vi "纳清DO电极校准.vi"() -> ()   [LabVIEW 2016, in "斯坦道多参数.lvlib"]
uses:
  <vilib>/Utility/miscctls.llb/LVPointTypeDef.ctl
  <vilib>/Analysis/NI_AALBase.lvlib
  <vilib>/ptbypt/NI_PtbyPt.lvlib
panel:
  out "标液2":string="饱和标准液"
  out "标液1":string="零点标准液"
  out "第二点信号值":dbl
  out "第一点信号值":dbl
  out "盐度":sgl format="%#.2f"
  out "大气压力":sgl format="%#.2f"
  out "饱和值":sgl format="%#.2f"
  out "报警信息":string
  out "通讯状态":string
  out "第二点校准值":dbl
  out "第一点校准值":dbl
  in  "校准停止":bool
  in  "校准启动":bool
  in  "校准模式":enum16{"两点校准", "单点校准"}(ring)=enum."单点校准"
  out "最小值":sgl format="%#.2f"
  out "最大值":sgl format="%#.2f"
  out "波形图表":dbl(graph) caption="历史曲线"
  out "mean":dbl caption="均值" format="%#.2f"
  out "standard deviation":dbl caption="标准差" format="%#.2f"
  out "变异系数":dbl format="%#.6f"
  out "测量值":sgl format="%#.2f"
  out "提示":string
  out "原始光强数值":sgl caption="信号值" format="%#.6f"
  out "温度":dbl format="%#.2f"
  # "DO电极设定"
  # "℃"
  # "mg/L"
  # "%"
  # "nA"
  # "kPa"
  # "ppt"
  # "请选择校准模式:"
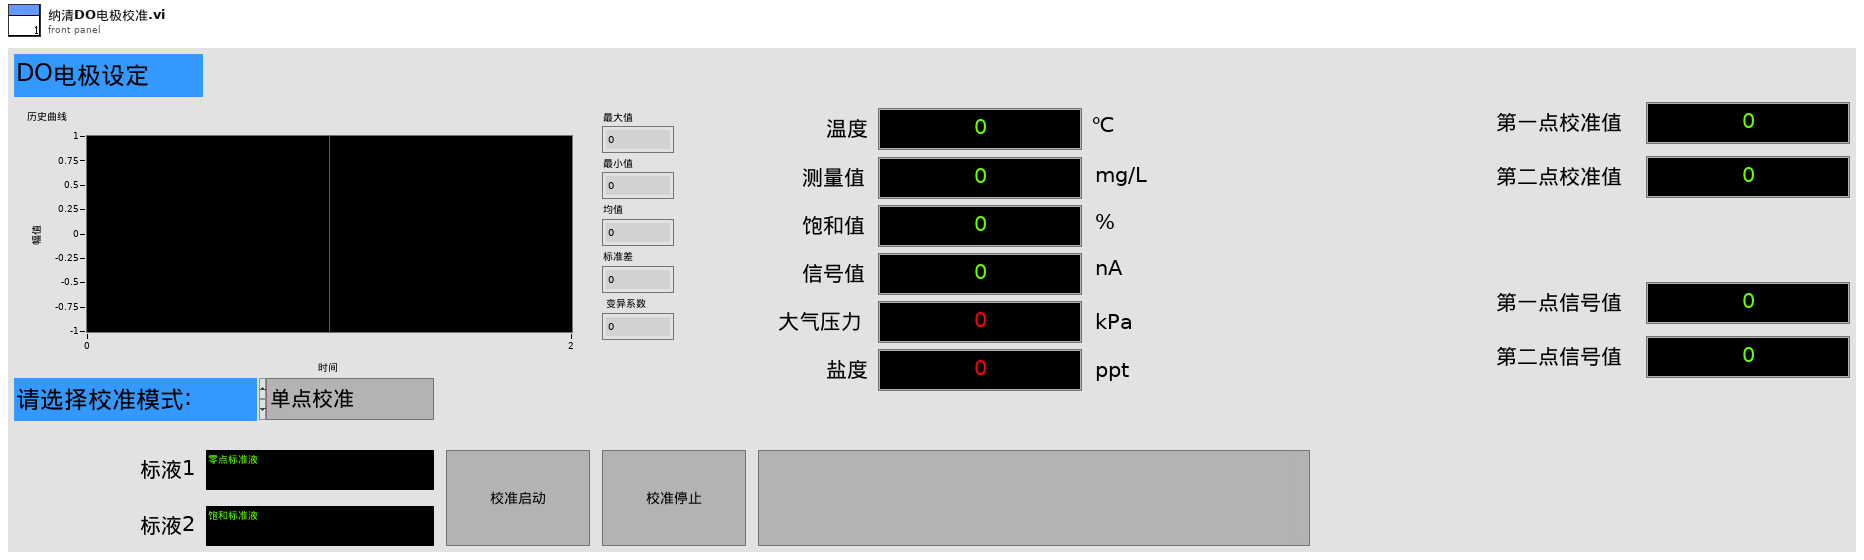
[diagram p1: front panel]
types:
  T1 = typedef "LVPointTypeDef.ctl" = cluster{"Horizontal":i16, "Vertical":i16}
  T2 = cluster{"报警码":u16, "溶解氧数值（mg/L）":sgl, "溶解氧数据（%）":sgl, "温度数据":sgl, "溶解氧原始信号 nA":sgl, "大气压力":sgl, "盐度":sgl, "0X0009_NC":string, "产品名称":string, "序列号":string, "硬件版本":string, "软件版本":string, "通讯地址":u16, "波特率":u16, "设备类型":u16, "0X0026_NC":string, "第一点原始数据":sgl, "第一点校准数据":sgl, "第二点原始数据":sgl, "第二点校准数据":sgl, "探头校准命令":u16, "温度校准参数":sgl, "温度校准命令":u16}
  T3 = enum8{"Enabled", "Disabled", "Disabled and Grayed Out"}
  T4 = cluster{"报警码":u16, "溶解氧数值（mg/L）":sgl, "溶解氧数据（%）":sgl, "温度数据":sgl, "溶解氧原始信号 nA":sgl, "大气压力":sgl, "盐度":sgl, "0X0009_NC":string, "产品名称":string, "序列号":string, "硬件版本":string, "软件版本":string, "通讯地址":u16, "波特率":u16, "设备类型":u16, "0X0026_NC":string, "第一点原始数据":sgl, "0X0033 NC":sgl, "第二点原始数据":sgl, "0X0037 NC":sgl, "探头校准命令":u16, "温度校准参数":sgl, "温度校准命令":u16}
  T5 = cluster{"ph":bool, "DO":bool, "Cond":bool, "Turb":bool, "叶绿素a":bool, "藻密度":bool, "ORP":bool}
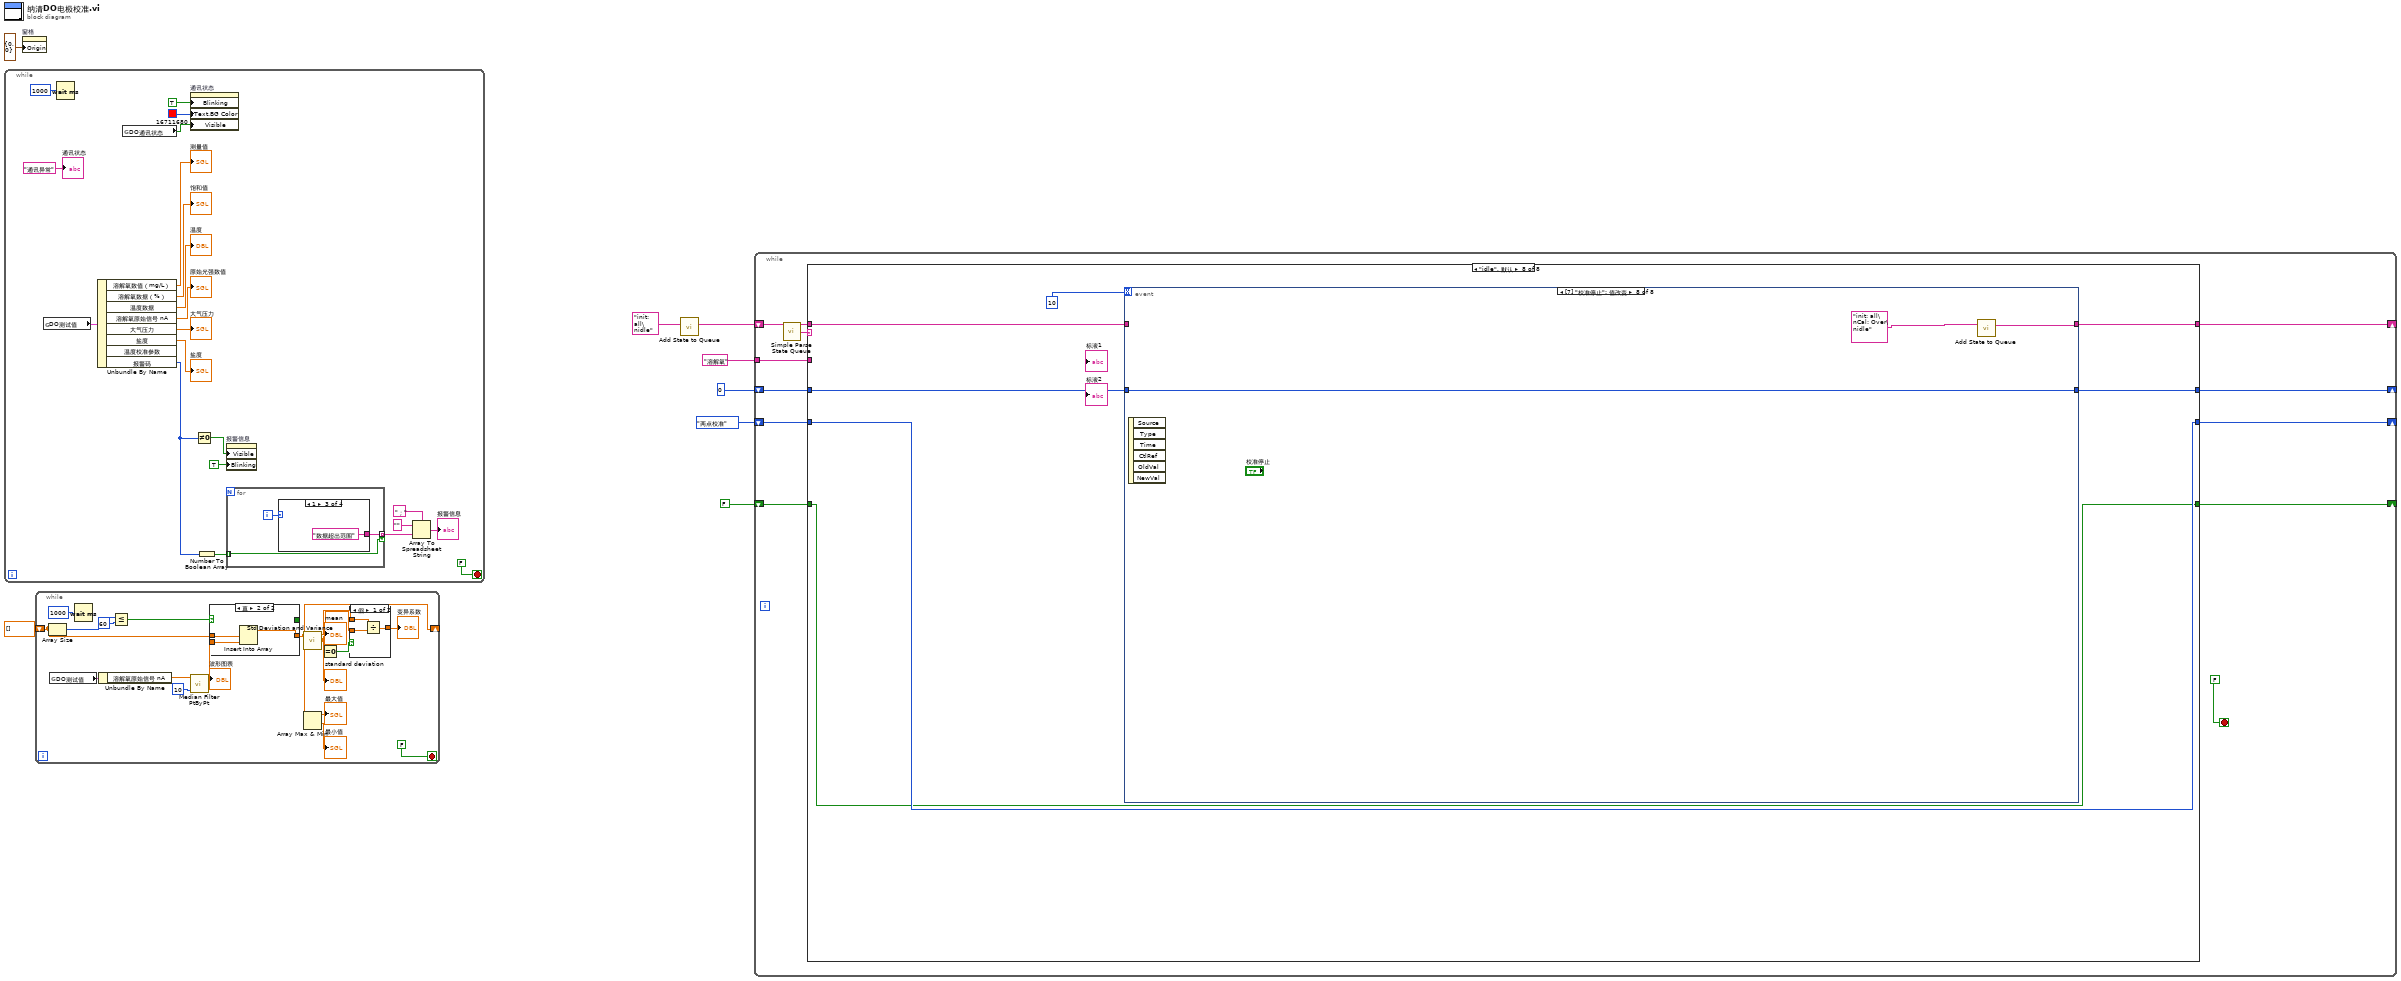
[diagram p0: block diagram]
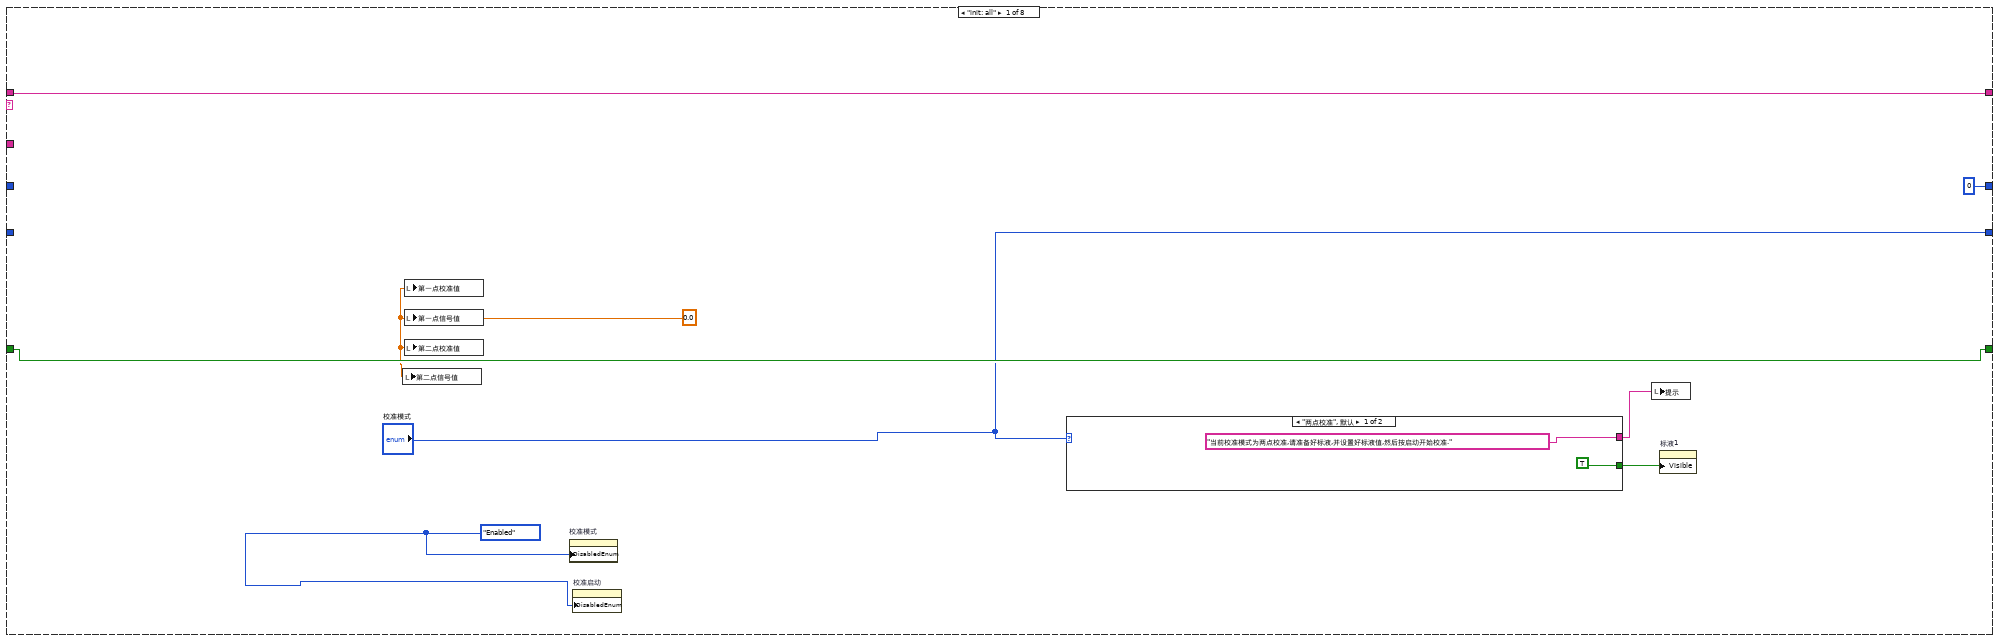
[diagram p2: hidden frame]
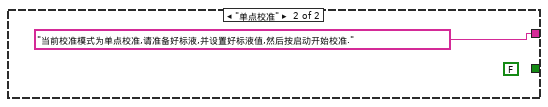
[diagram p3: hidden frame]
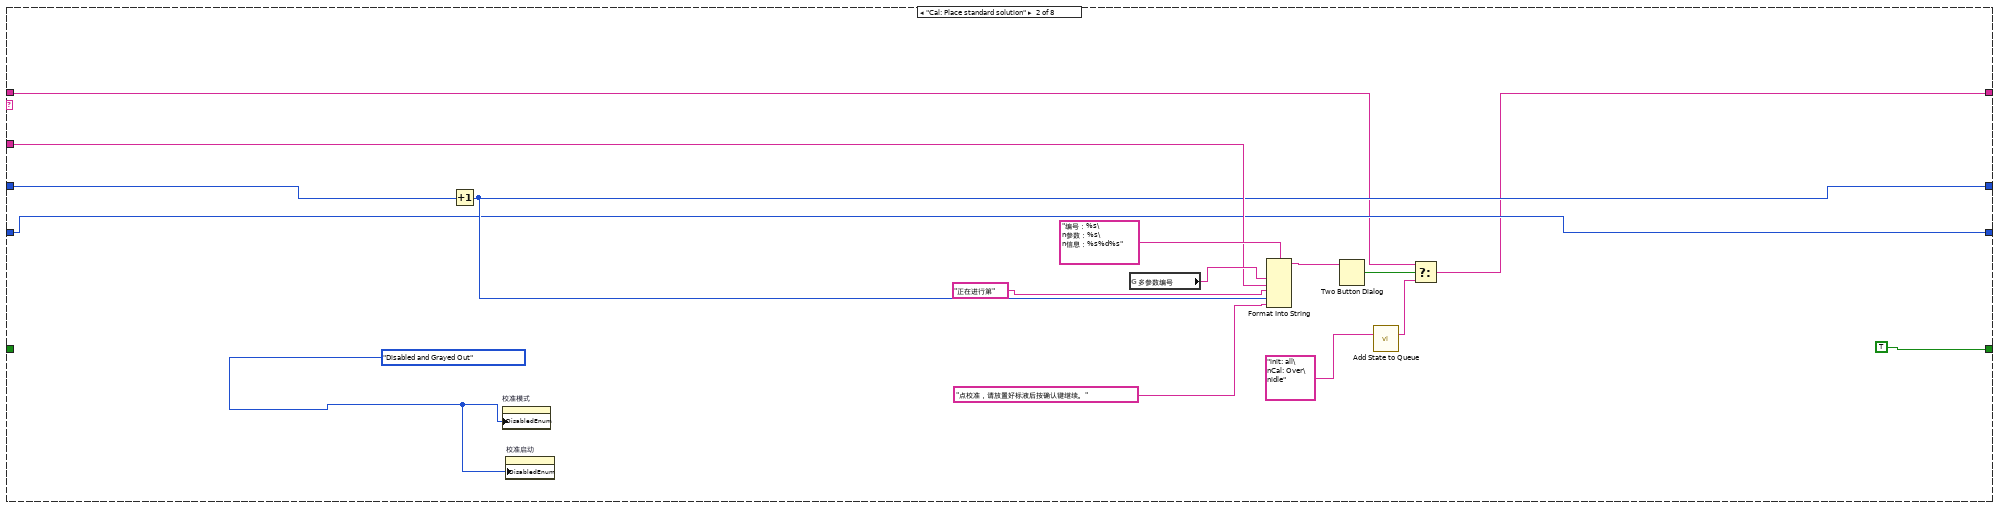
[diagram p4: hidden frame]
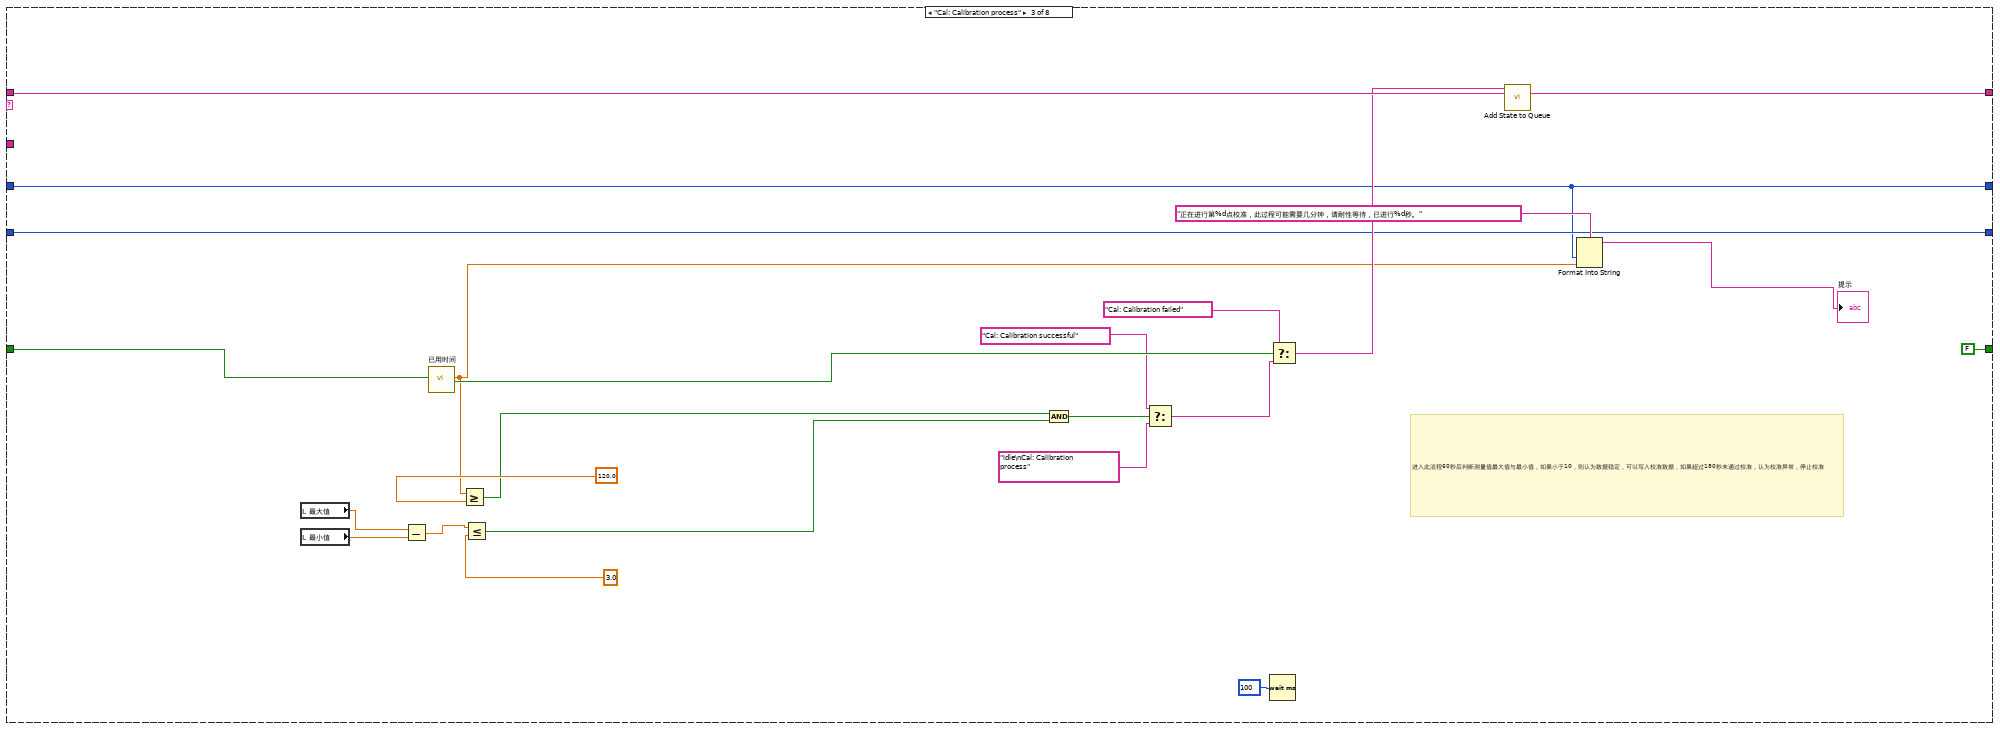
[diagram p5: hidden frame]
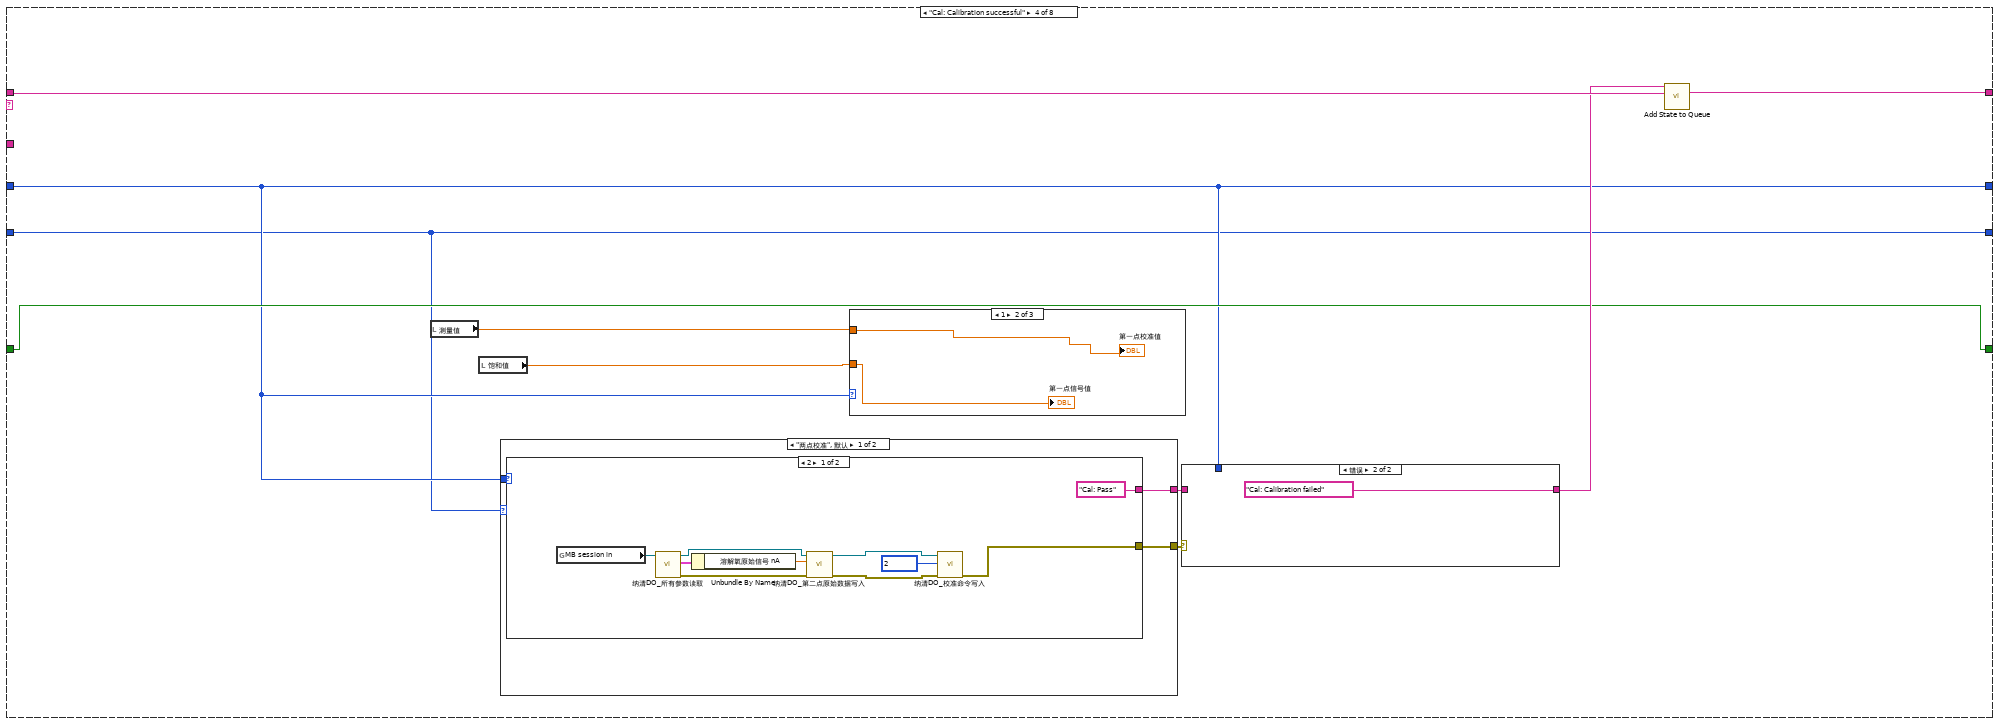
[diagram p6: hidden frame]
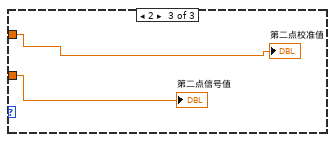
[diagram p8: hidden frame]
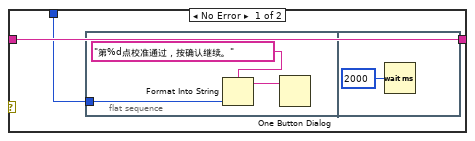
[diagram p9: hidden frame]
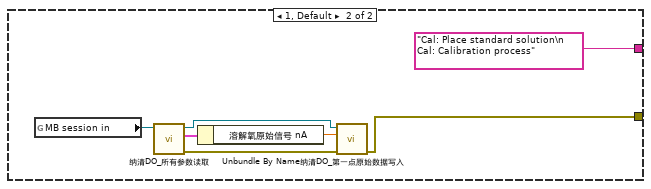
[diagram p10: hidden frame]
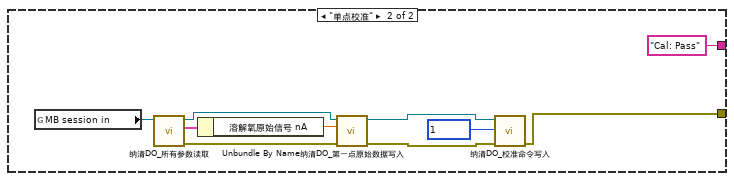
[diagram p11: hidden frame]
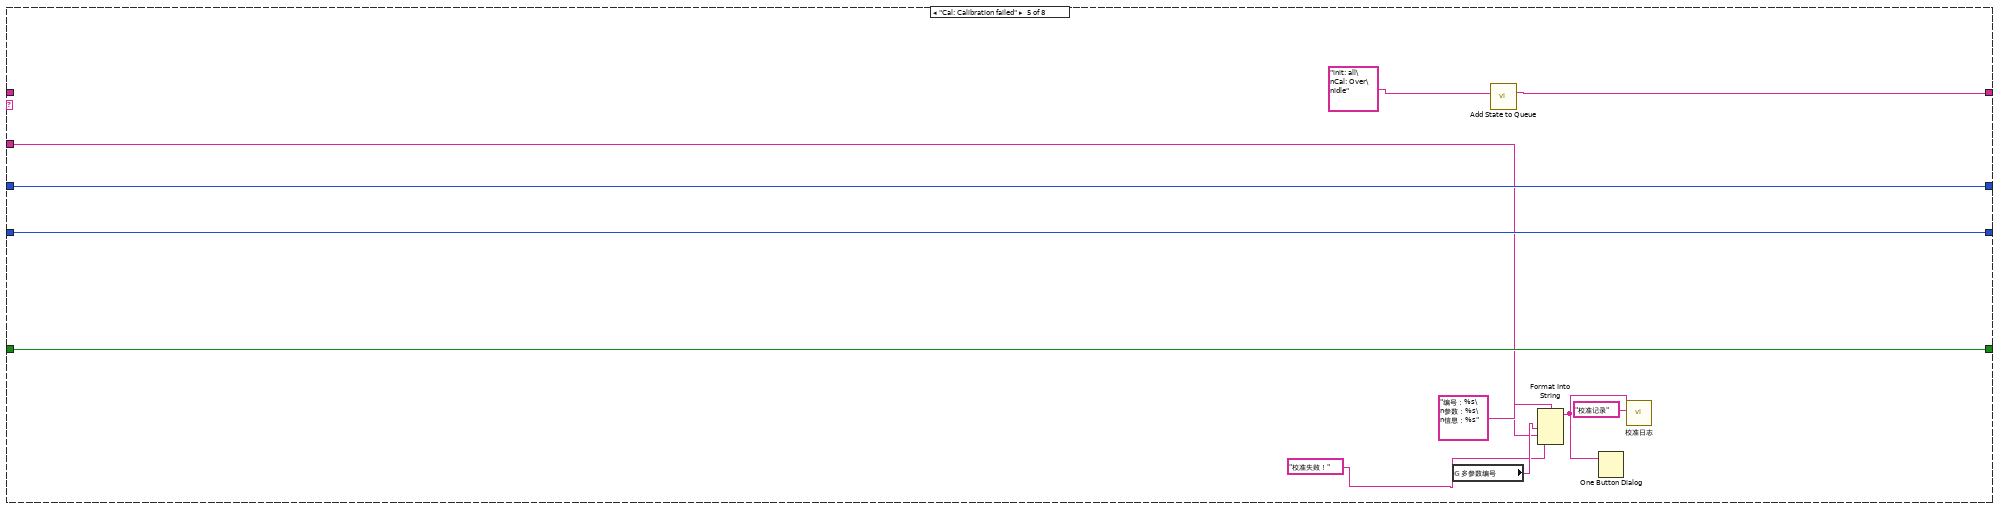
[diagram p12: hidden frame]
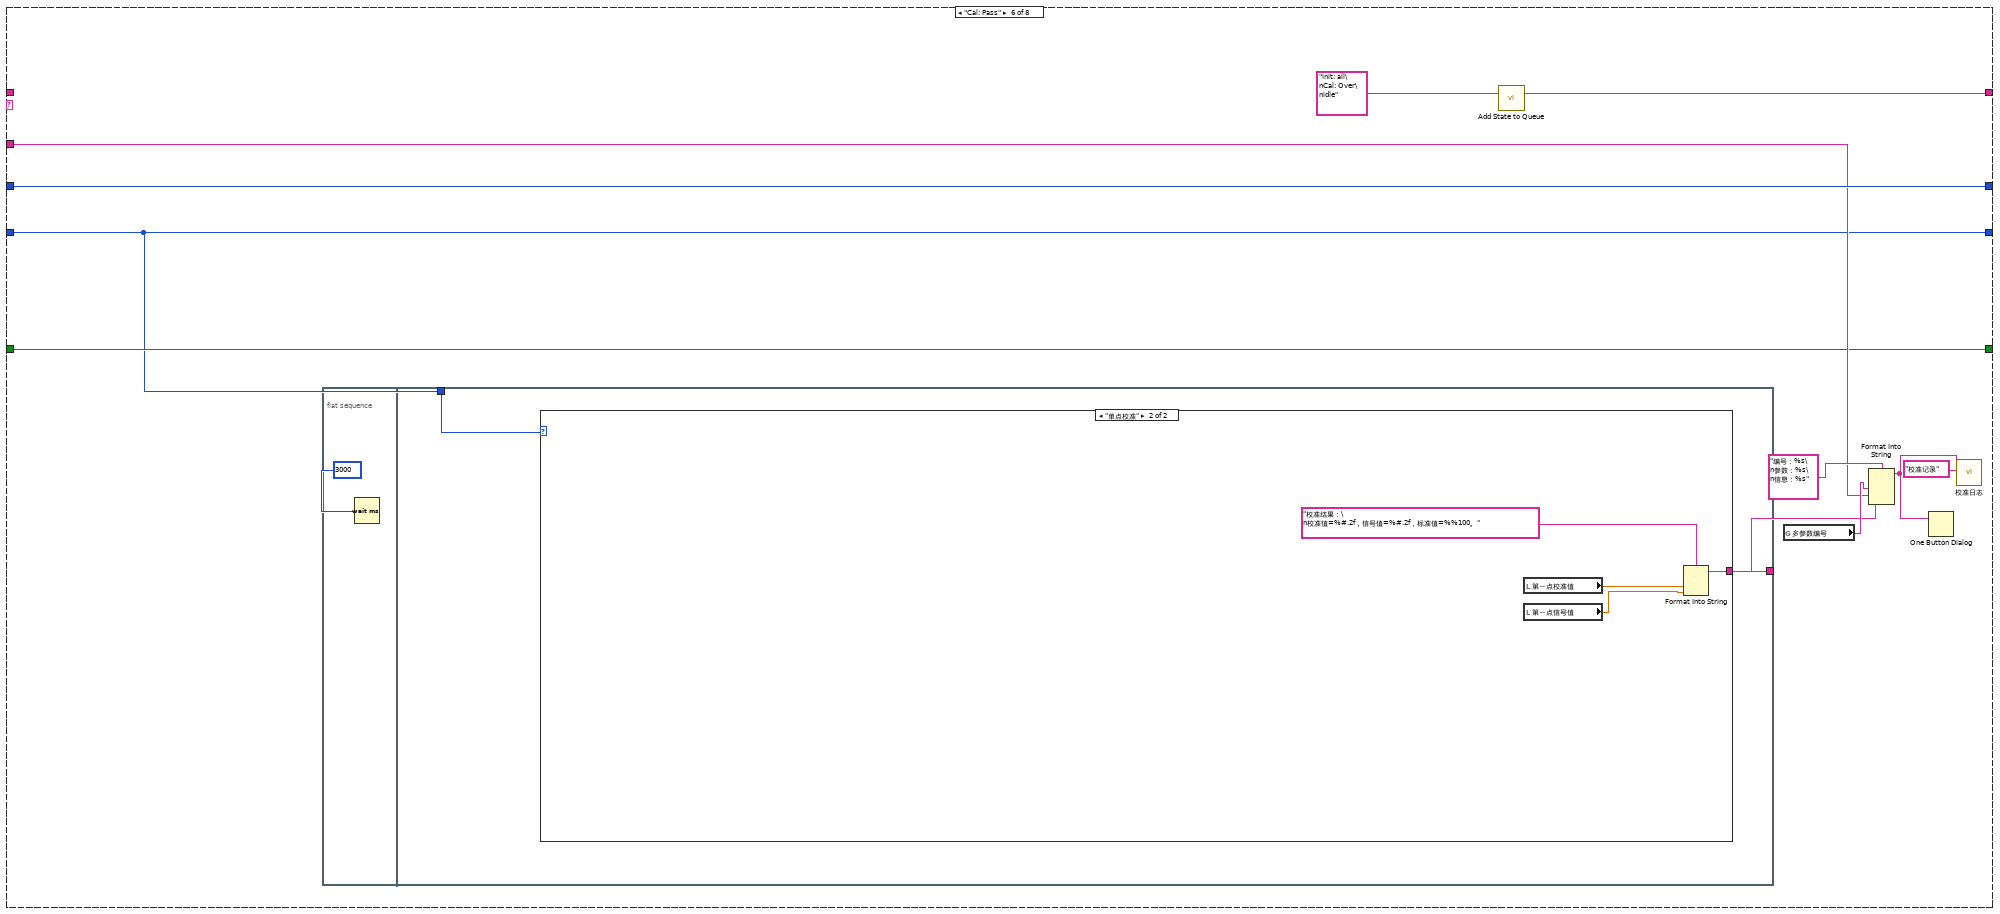
[diagram p13: hidden frame]
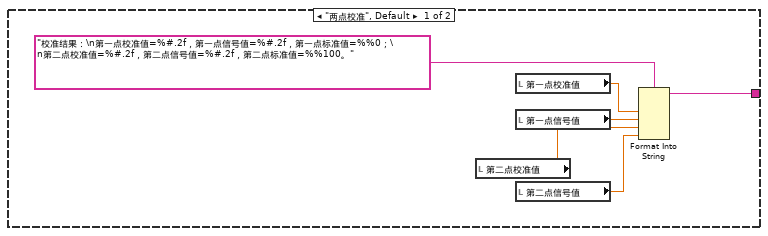
[diagram p14: hidden frame]
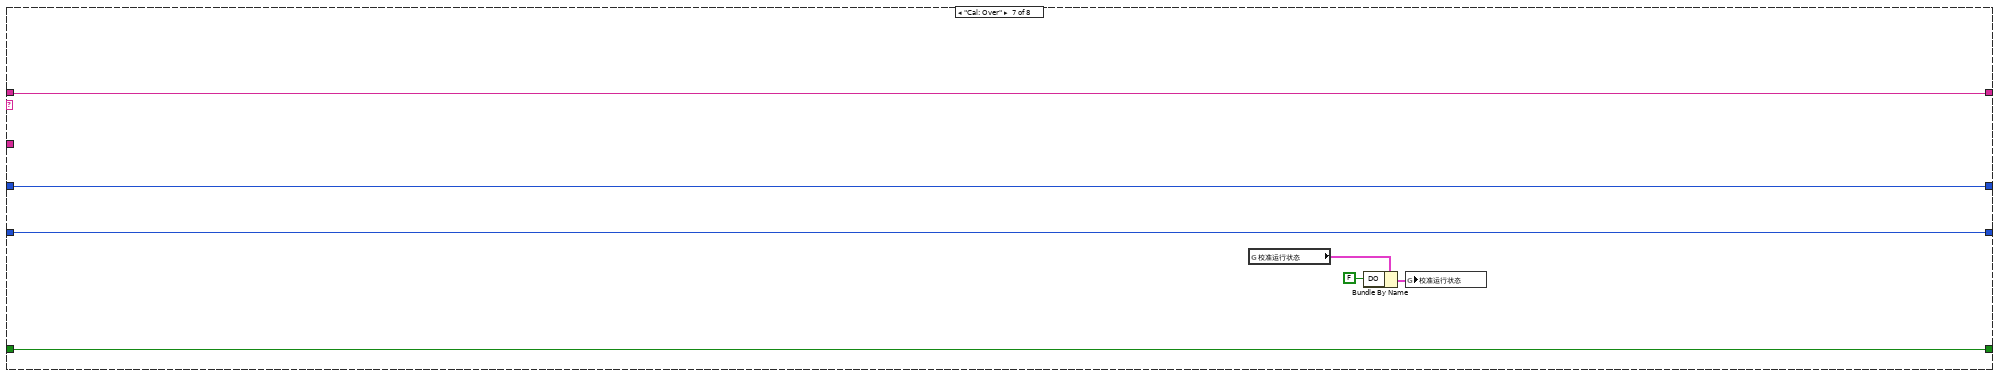
[diagram p15: hidden frame]
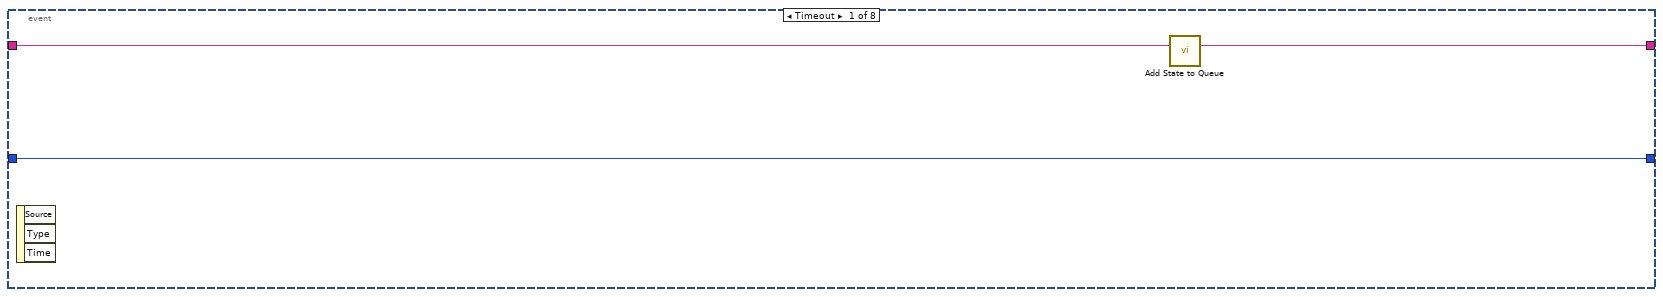
[diagram p16: hidden frame]
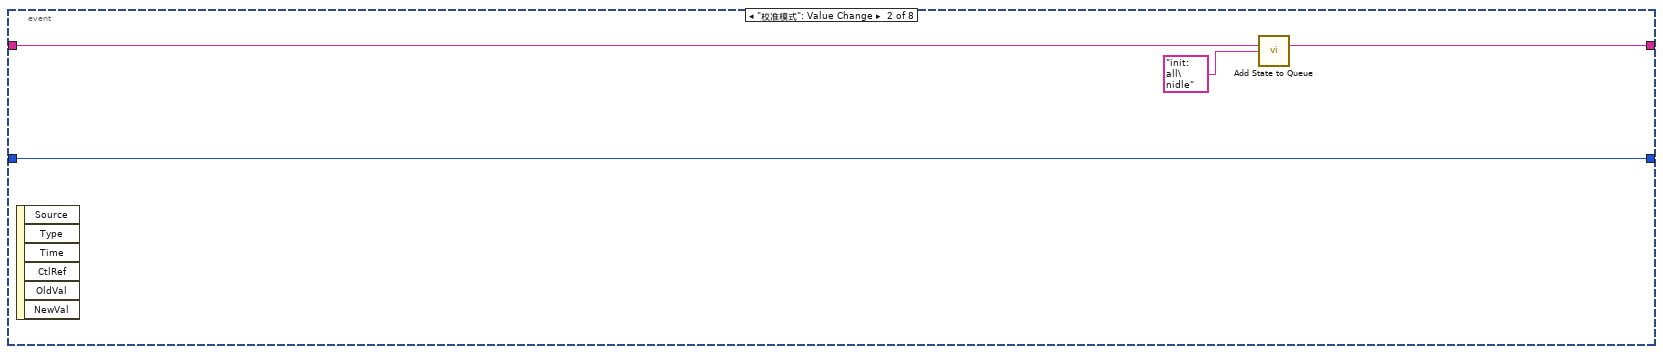
[diagram p17: hidden frame]
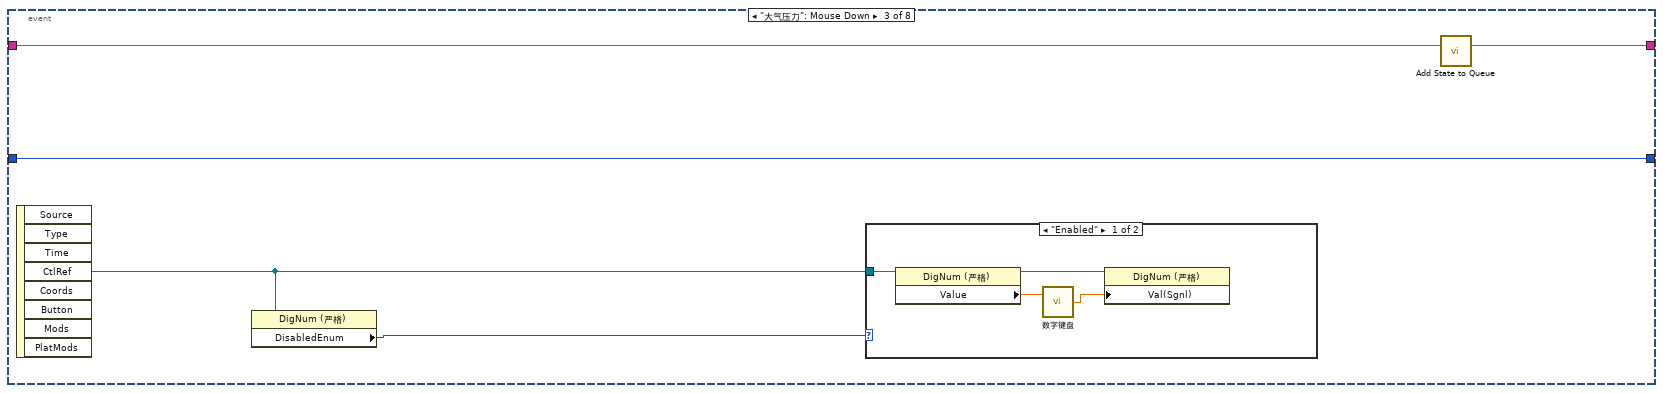
[diagram p18: hidden frame]
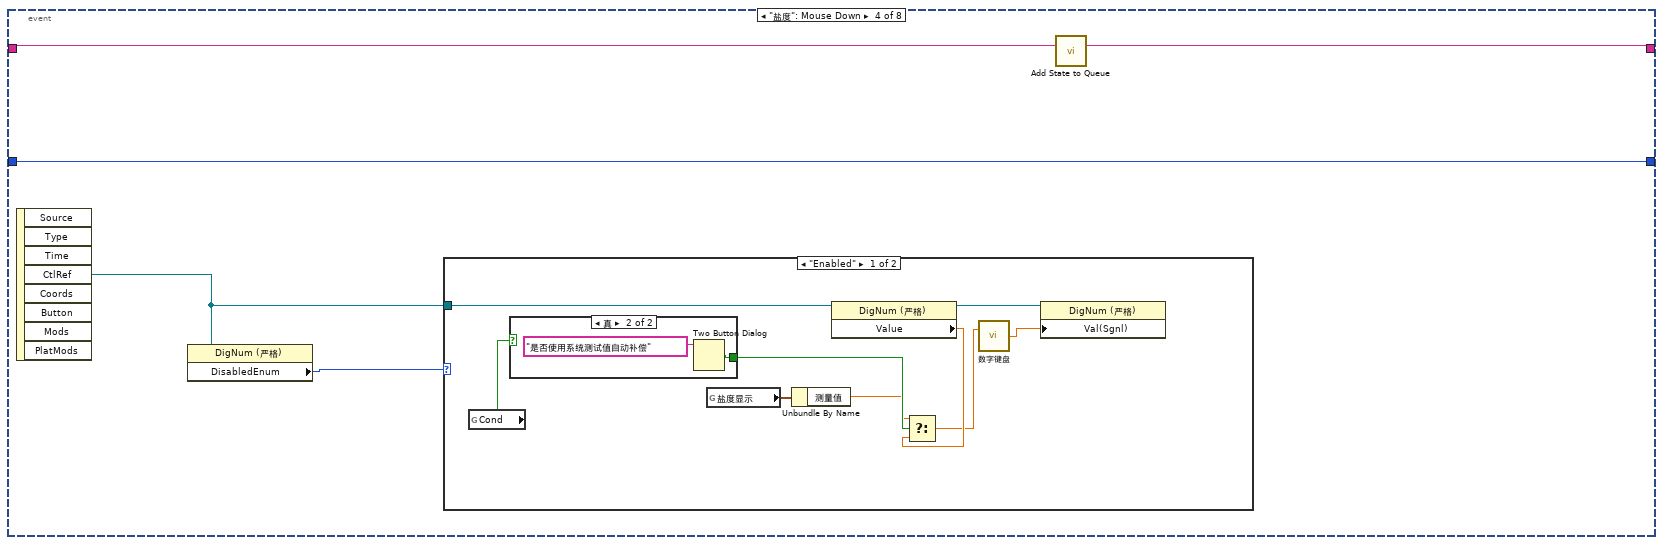
[diagram p20: hidden frame]
diagram:
  n1 = while {
    stop <- FALSE stop-if-true
    n2 = global read "纳清过程全局变量.vi" "DO测试值"() -> (w27:T2)
    n3 = Wait (ms)(milliseconds to wait=u32 1000 ("等待时间（毫秒）")) -> ()  [unwired: 1 out]
    n4 = Unbundle By Name(w27) -> ("溶解氧数值（mg/L）"=→"测量值":sgl, "溶解氧数据（%）"=→"饱和值":sgl, "温度数据"=→"温度":sgl, "溶解氧原始信号 nA"=→"原始光强数值":sgl, "大气压力"=→"大气压力":sgl, "盐度"=→"盐度":sgl, "报警码"=w14:u16)  [unwired: 1 out]
    n5 = global read "多参数全局变量.vi" "DO通讯状态"() -> (w20:bool)
    n6 = property on="通讯状态" class="Str"("Blinking"=TRUE ("闪烁"), "Text.BG Color"=u32 16711680, "Visible"=w20) -> ()  [unwired: 2 in, 2 out]
    n7 = Not Equal To 0?(x=w14) -> (x != 0?=w13:bool)
    n8 = Number To Boolean Array(number=w14) -> (Boolean array=w19:bool[])
    n9 = property on="报警信息" class="Str"("Visible"=w13, "Blinking"=TRUE ("闪烁")) -> ()  [unwired: 2 in, 2 out]
    n10 = for {
      tunnel: w19 -> [w30] mode=indexing
      tunnel: [w31] -> w18 mode=indexing if=w30
      i -> [w32]
      n11 = case shown="1" w32 {
        tunnel: [_ "温度超出范围" "数据超出范围" "温度传感器故障"] -> w31
        frame Default {
        }
        frame 0 {
        }
        frame 1 {
        }
        frame 8 {
        }
      }
    }
    n12 = Array To Spreadsheet String(delimiter (Tab)="；" ("分隔符(Tab)"), array=w18, 3:"" ("格式字符串")) -> (spreadsheet string=→"报警信息":string)
    "通讯状态" <- "通讯异常" ("当前串口")
  }
  n13 = property on="窗格" class="Pane"("Origin"=T1 {"Horizontal"=0, "Vertical"=0} ("原点")) -> ()  [unwired: 2 in, 2 out]
  n14 = while {
    shift-right: [w42] -> _
    shift-left: sgl[] [] -> [w48]
    stop <- FALSE stop-if-true
    n15 = Array Size(array=w48) -> (size(s)=w50:i32)
    n16 = global read "纳清过程全局变量.vi" "DO测试值"() -> (w39:T2)
    n17 = Wait (ms)(milliseconds to wait=u32 1000 ("等待时间（毫秒）")) -> ()  [unwired: 1 out]
    n18 = Unbundle By Name(w39) -> ("溶解氧原始信号 nA"=w37:sgl)
    n19 = Less Or Equal?(x=w50, y=60) -> (x <= y?=w49:bool)
    n20 = call <vilib>:"Median Filter PtByPt.vi"("rank"=10, "x"=w37) -> ("Filtered x"=w36:dbl)  [unwired: 2 in, 1 out]
    "波形图表" <- w36
    n21 = case shown="真" w49 {
      tunnel: w48 -> [w61 w64]
      tunnel: w36 -> [w59 w63]
      tunnel: [w57 w62] -> w42
      tunnel: [TRUE _] -> _
      frame False {
        n22 = Replace Array Subset(array=w61, new element=w59) -> (w60:sgl[])  [unwired: 1 in]
        n23 = Rotate 1D Array(1:w60, 2:-1 ("n")) -> (0:w57:sgl[])
      }
      frame True {
        n24 = Insert Into Array(array=w64, new element=w63) -> (w62:sgl[])  [unwired: 1 in]
      }
    }
    n25 = call <vilib>:"Std Deviation and Variance.vi"("X"=w42) -> ("mean"=w46:dbl, "standard deviation"=w45:dbl)  [unwired: 1 in, 1 out]
    "mean" <- w46
    "standard deviation" <- w45
    n26 = Array Max & Min(array=w42) -> (max value=→"最大值":sgl, min value=→"最小值":sgl)  [unwired: 2 out]
    n27 = Equal To 0?(x=w46) -> (x = 0?=w47:bool)
    n28 = case shown="假" w47 {
      tunnel: w45 -> [w55 _]
      tunnel: [w54 _] -> w44
      tunnel: w46 -> [w53 _]
      frame False {
        n29 = Divide(x=w55, y=w53) -> (x/y=w54:dbl)
      }
      frame True {
      }
    }
    "变异系数" <- w44
  }
  n30 = call "Add State to Queue.vi"("State(s) In (\"\")"="init: all\nidle" ("State(s) In (\"\")")) -> ("States Out"=w5:string)  [unwired: 14 in]
  n31 = while {
    shift-right: [w72] -> _
    shift-left: w5 -> [w76]
    shift-right: [w69] -> _
    shift-left: 0 -> [w71]
    tunnel: "溶解氧" ("State(s) In (\"\")") -> [w70]
    shift-right: [w67] -> _
    shift-left: enum16{"两点校准", "单点校准"}."两点校准" ("校准模式") -> [w68]
    shift-right: [w65] -> _
    shift-left: FALSE -> [w66]
    stop <- FALSE stop-if-true
    n32 = call "Simple Parse State Queue.vi"("State Queue"=w76) -> ("Remain States"=w73:string, "Next State"=w74:string)  [unwired: 13 in]
    n33 = case shown="\"idle\", 默认" w74 {
      tunnel: w73 -> [w84 w91 w122 w135 _ _ w220 w227]
      tunnel: [w84 w90 w121 w134 w186 w191 w220 w226] -> w72
      tunnel: w71 -> [_ w99 w106 w129 w189 w200 w219 w224]
      tunnel: w70 -> [_ w100 _ _ w180 w196 _ _]
      tunnel: [0 w97 w106 w129 w189 w200 w219 w225] -> w69
      tunnel: w68 -> [_ w96 w107 w128 w188 w192 w218 w223]
      tunnel: ["校准模式" w96 w107 w128 w188 w192 w218 w223] -> w67
      tunnel: w66 -> [w81 _ w109 w130 w187 w195 w217 w221]
      tunnel: [w81 TRUE FALSE w130 w187 w195 w217 w221] -> w65
      frame "init: all" {
        w78 = T3."Enabled" ("禁用")
        w80 = 0.0 ("第一点校准值")
        n34 = local write "第二点信号值"(w80) -> ()
        n35 = local write "第一点校准值"(w80) -> ()
        n36 = local write "第一点信号值"(w80) -> ()
        n37 = local write "第二点校准值"(w80) -> ()
        n38 = property on="校准模式" class="Enum (严格)"("DisabledEnum"=w78) -> ()  [unwired: 2 in, 2 out]
        n39 = property on="校准启动" class="Bool"("DisabledEnum"=w78) -> ()  [unwired: 2 in, 2 out]
        n40 = case shown="\"两点校准\", 默认" "校准模式" {
          tunnel: ["当前校准模式为两点校准,请准备好标液,并设置好标液值,然后按启动开始校准." ("提示") "当前校准模式为单点校准,请准备好标液,并设置好标液值,然后按启动开始校准." ("提示")] -> w83
          tunnel: [TRUE ("可见") _] -> w77
          frame "两点校准", Default {
          }
          frame "单点校准" {
            (unwired) FALSE ("可见")
          }
        }
        n41 = local write "提示"(w83) -> ()
        n42 = property on="标液1" class="Str"("Visible"=w77) -> ()  [unwired: 2 in, 2 out]
      }
      frame "Cal: Place standard solution" {
        w89 = T3."Disabled and Grayed Out" ("禁用")
        n43 = Increment(x=w99) -> (x+1=w97:i32)
        n44 = property on="校准模式" class="Enum (严格)"("DisabledEnum"=w89) -> ()  [unwired: 2 in, 2 out]
        n45 = property on="校准启动" class="Bool"("DisabledEnum"=w89) -> ()  [unwired: 2 in, 2 out]
        n46 = global read "多参数全局变量.vi" "多参数编号"() -> (w102:string)
        n47 = Format Into String(format string="编号：%s\n参数：%s\n信息：%s%d%s" ("格式字符串"), w102, w100, "正在进行第" ("消息"), w97, "点校准，请放置好标液后按确认键继续。" ("消息")) -> (resulting string=w94:string)  [unwired: 2 in, 1 out]
        n48 = Two Button Dialog(message=w94) -> (T button?=w93:bool)  [unwired: 2 in]
        n49 = call "Add State to Queue.vi"("State(s) In (\"\")"="init: all\nCal: Over\nidle" ("State(s) In (\"\")")) -> ("States Out"=w92:string)  [unwired: 14 in]
        n50 = Select(t=w91, s=w93, f=w92) -> (s? t:f=w90:string)
      }
      frame "Cal: Calibration process" {
        # "进入此流程60秒后判断测量值最大值与最小值，如果小于10，则认为数据稳定，可以写入校准数据，如果超过180秒未通过校准，认为校准异常，停止校准"
        n51 = local read "最大值"() -> (w126:sgl)
        n52 = local read "最小值"() -> (w125:sgl)
        n53 = Subtract(x=w126, y=w125) -> (x-y=w127:sgl)
        n54 = call "已用时间"("Reset"=w109) -> ("Elapsed Time (s)"=w105:dbl, "Time has Elapsed"=w123:bool)  [unwired: 11 in, 6 out]
        n55 = Greater Or Equal?(x=w105, y=120.0) -> (x >= y?=w118:bool)
        n56 = Less Or Equal?(x=w127, y=3.0) -> (x <= y?=w114:bool)
        n57 = And(x=w118, y=w114) -> (x .and. y?=w115:bool)
        n58 = Select(t="Cal: Calibration successful" ("State(s) In (\"\")"), s=w115, f="idle\nCal: Calibration process" ("State(s) In (\"\")")) -> (s? t:f=w113:string)
        n59 = Wait (ms)(milliseconds to wait=u32 100 ("等待时间（毫秒）")) -> ()  [unwired: 1 out]
        n60 = Select(t="Cal: Calibration failed" ("State(s) In (\"\")"), s=w123, f=w113) -> (s? t:f=w112:string)
        n61 = call "Add State to Queue.vi"("State(s) In Front (\"\")"=w112, "State(s) In (\"\")"=w122) -> ("States Out"=w121:string)  [unwired: 13 in]
        n62 = Format Into String(format string="正在进行第%d点校准，此过程可能需要几分钟，请耐性等待，已进行%d秒。" ("格式字符串"), w106, w105) -> (resulting string=→"提示":string)  [unwired: 2 in, 1 out]
      }
      frame "Cal: Calibration successful" {
        n63 = local read "测量值"() -> (w131:sgl)
        n64 = local read "饱和值"() -> (w132:sgl)
        n65 = case shown="\"两点校准\", 默认" w128 {
          tunnel: [w151 w169] -> w137
          tunnel: [w150 "Cal: Pass" ("State(s) In (\"\")")] -> w136
          tunnel: w129 -> [w149 _]
          frame "两点校准", Default {
            n66 = case shown="2" w149 {
              tunnel: [w153 w162] -> w151
              tunnel: ["Cal: Pass" ("State(s) In (\"\")") "Cal: Place standard solution\n Cal: Calibration process" ("State(s) In (\"\")")] -> w150
              frame 2 {
                n67 = global read "多参数全局变量.vi" "MB session in"() -> (w158:refnum<class "MB_Master.lvclass">)
                n68 = call "纳清DO_所有参数读取.vi"("MB session in"=w158) -> ("error out"=w160:errorcluster, "输出值"=w157:T4, "MB session out"=w159:refnum<class "MB_Master.lvclass">)  [unwired: 8 in]
                n69 = Unbundle By Name(w157) -> ("溶解氧原始信号 nA"=w156:sgl)
                n70 = call "纳清DO_第二点原始数据写入.vi"("error in (no error)"=w160, "数值"=w156, "MB session in"=w159) -> ("error out"=w155:errorcluster, "MB session out"=w154:refnum<class "MB_Master.lvclass">)  [unwired: 7 in]
                n71 = call "纳清DO_校准命令写入.vi"("error in (no error)"=w155, "数值"=u16 2 ("starting address"), "MB session in"=w154) -> ("error out"=w153:errorcluster)  [unwired: 7 in, 1 out]
              }
              frame 1, Default {
                n72 = global read "多参数全局变量.vi" "MB session in"() -> (w165:refnum<class "MB_Master.lvclass">)
                n73 = call "纳清DO_所有参数读取.vi"("MB session in"=w165) -> ("error out"=w167:errorcluster, "输出值"=w164:T4, "MB session out"=w166:refnum<class "MB_Master.lvclass">)  [unwired: 8 in]
                n74 = Unbundle By Name(w164) -> ("溶解氧原始信号 nA"=w163:sgl)
                n75 = call "纳清DO_第一点原始数据写入.vi"("error in (no error)"=w167, "数值"=w163, "MB session in"=w166) -> ("error out"=w162:errorcluster)  [unwired: 7 in, 1 out]
              }
            }
          }
          frame "单点校准" {
            n76 = global read "多参数全局变量.vi" "MB session in"() -> (w175:refnum<class "MB_Master.lvclass">)
            n77 = call "纳清DO_所有参数读取.vi"("MB session in"=w175) -> ("error out"=w177:errorcluster, "输出值"=w174:T4, "MB session out"=w176:refnum<class "MB_Master.lvclass">)  [unwired: 8 in]
            n78 = Unbundle By Name(w174) -> ("溶解氧原始信号 nA"=w173:sgl)
            n79 = call "纳清DO_第一点原始数据写入.vi"("error in (no error)"=w177, "数值"=w173, "MB session in"=w176) -> ("error out"=w172:errorcluster, "MB session out"=w171:refnum<class "MB_Master.lvclass">)  [unwired: 7 in]
            n80 = call "纳清DO_校准命令写入.vi"("error in (no error)"=w172, "数值"=u16 1 ("starting address"), "MB session in"=w171) -> ("error out"=w169:errorcluster)  [unwired: 7 in, 1 out]
          }
        }
        n81 = case shown="1" w129 {
          tunnel: w132 -> [_ w139 w141]
          tunnel: w131 -> [_ w138 w140]
          frame 0, Default {
          }
          frame 1 {
            "第一点信号值" <- w139
            "第一点校准值" <- w138
          }
          frame 2 {
            "第二点信号值" <- w141
            "第二点校准值" <- w140
          }
        }
        n82 = case shown="错误" w137 {
          tunnel: w136 -> [w143 _]
          tunnel: [w143 "Cal: Calibration failed" ("State(s) In (\"\")")] -> w133
          tunnel: w129 -> [w142 _]
          frame No Error {
            n83 = flat-sequence {
              tunnel: w142 -> [w144]
              frame #0 {
                n84 = Format Into String(format string="第%d点校准通过，按确认继续。" ("格式字符串"), w144) -> (resulting string=w146:string)  [unwired: 2 in, 1 out]
                n85 = One Button Dialog(message=w146) -> ()  [unwired: 1 in, 1 out]
              }
              frame #1 {
                n86 = Wait (ms)(milliseconds to wait=u32 2000 ("等待时间（毫秒）")) -> ()  [unwired: 1 out]
              }
            }
          }
          frame Error {
          }
        }
        n87 = call "Add State to Queue.vi"("State(s) In Front (\"\")"=w133, "State(s) In (\"\")"=w135) -> ("States Out"=w134:string)  [unwired: 13 in]
      }
      frame "Cal: Calibration failed" {
        n88 = global read "多参数全局变量.vi" "多参数编号"() -> (w183:string)
        n89 = call "Add State to Queue.vi"("State(s) In (\"\")"="init: all\nCal: Over\nidle" ("State(s) In (\"\")")) -> ("States Out"=w186:string)  [unwired: 14 in]
        n90 = Format Into String(format string="编号：%s\n参数：%s\n信息：%s" ("格式字符串"), w183, w180, "校准失败！" ("消息")) -> (resulting string=w182:string)  [unwired: 2 in, 1 out]
        n91 = One Button Dialog(message=w182) -> ()  [unwired: 1 in, 1 out]
        n92 = call "校准日志.vi"("table"="校准记录", "日志信息"=w182) -> ()  [unwired: 9 in, 1 out]
      }
      frame "Cal: Pass" {
        n93 = flat-sequence {
          tunnel: [w203] -> w193
          tunnel: w192 -> [w202]
          frame #0 {
            n94 = Wait (ms)(milliseconds to wait=u32 3000 ("等待时间（毫秒）")) -> ()  [unwired: 1 out]
          }
          frame #1 {
            n95 = case shown="\"单点校准\"" w202 {
              tunnel: [w209 w213] -> w203
              frame "两点校准", Default {
                n96 = local read "第二点校准值"() -> (w205:dbl)
                n97 = local read "第一点校准值"() -> (w207:dbl)
                n98 = local read "第一点信号值"() -> (w208:dbl)
                n99 = local read "第二点信号值"() -> (w204:dbl)
                n100 = Format Into String(format string="校准结果：\n第一点校准值=%#.2f，第一点信号值=%#.2f，第一点标准值=%%0；\n第二点校准值=%#.2f，第二点信号值=%#.2f，第二点标准值=%%100。" ("提示"), w207, w208, w205, w204) -> (resulting string=w209:string)  [unwired: 2 in, 1 out]
              }
              frame "单点校准" {
                n101 = local read "第一点校准值"() -> (w212:dbl)
                n102 = local read "第一点信号值"() -> (w210:dbl)
                n103 = Format Into String(format string="校准结果：\n校准值=%#.2f，信号值=%#.2f，标准值=%%100。" ("提示"), w212, w210) -> (resulting string=w213:string)  [unwired: 2 in, 1 out]
              }
            }
          }
        }
        n104 = call "Add State to Queue.vi"("State(s) In (\"\")"="init: all\nCal: Over\nidle" ("State(s) In (\"\")")) -> ("States Out"=w191:string)  [unwired: 14 in]
        n105 = global read "多参数全局变量.vi" "多参数编号"() -> (w197:string)
        n106 = Format Into String(format string="编号：%s\n参数：%s\n信息：%s" ("格式字符串"), w197, w196, w193) -> (resulting string=w194:string)  [unwired: 2 in, 1 out]
        n107 = One Button Dialog(message=w194) -> ()  [unwired: 1 in, 1 out]
        n108 = call "校准日志.vi"("table"="校准记录", "日志信息"=w194) -> ()  [unwired: 9 in, 1 out]
      }
      frame "Cal: Over" {
        n109 = global read "多参数全局变量.vi" "校准运行状态"() -> (w215:T5)
        n110 = Bundle By Name(cluster=w215, "DO"=FALSE) -> (w216:T5)
        n111 = global write "多参数全局变量.vi" "校准运行状态"(w216) -> ()
      }
      frame "idle", Default {
        n112 = event shown="[7] \"校准停止\": 值改变" {
          selector: _ -> [_ _ _ _ _ _ _ _]
          dyn-events: _ -> [_ _ _ _ _ _ _ _]
          timeout: 10 -> [_ _ _ _ _ _ _ _]
          tunnel: w227 -> [w230 w234 w237 w244 w260 w265 w276 _]
          tunnel: [w229 w233 w238 w248 w264 w269 w275 w278] -> w226
          tunnel: [w228 w231 w239 w247 w263 w268 w273 w279] -> w225
          tunnel: w224 -> [w228 w231 w239 w247 w263 w268 w273 w279]
          event Timeout {
            n113 = event-data() -> ()  [unwired: 1 in, 3 out]
            n114 = call "Add State to Queue.vi"("State(s) In (\"\")"=w230) -> ("States Out"=w229:string)  [unwired: 14 in]
          }
          event "校准模式": Value Change {
            n115 = event-data() -> ()  [unwired: 1 in, 6 out]
            n116 = call "Add State to Queue.vi"("State(s) In (\"\")"=w234, "State(s) At Back (\"\")"="init: all\nidle" ("State(s) In (\"\")")) -> ("States Out"=w233:string)  [unwired: 13 in]
          }
          event "大气压力": Mouse Down {
            n117 = event-data() -> ("CtlRef"=w236:refnum<vi>)  [unwired: 1 in, 7 out]
            n118 = property class="DigNum (严格)"(reference=w236) -> ("DisabledEnum"=w235:T3)  [unwired: 1 in, 2 out]
            n119 = case shown="\"Enabled\"" w235 {
              tunnel: w236 -> [w243 _]
              frame "Enabled" {
                n120 = property class="DigNum (严格)"(reference=w243) -> (reference out=w240:refnum<vi>, "Value"=w241:sgl)  [unwired: 1 in, 1 out]
                n121 = call "数字键盘.vi"("OldNumber"=w241) -> ("NewNumber"=w242:dbl)  [unwired: 1 in]
                n122 = property class="DigNum (严格)"(reference=w240, "Val(Sgnl)"=w242) -> ()  [unwired: 1 in, 2 out]
              }
              frame "Disabled", Default {
              }
            }
            n123 = call "Add State to Queue.vi"("State(s) In (\"\")"=w237) -> ("States Out"=w238:string)  [unwired: 14 in]
          }
          event "盐度": Mouse Down {
            n124 = event-data() -> ("CtlRef"=w245:refnum<vi>)  [unwired: 1 in, 7 out]
            n125 = property class="DigNum (严格)"(reference=w245) -> ("DisabledEnum"=w246:T3)  [unwired: 1 in, 2 out]
            n126 = case shown="\"Enabled\"" w246 {
              tunnel: w245 -> [w257 _]
              frame "Enabled" {
                n127 = global read "断电保存变量.vi" "Cond"() -> (w249:bool)
                n128 = case shown="真" w249 {
                  tunnel: [_ w258] -> w254
                  frame False {
                  }
                  frame True {
                    n129 = Two Button Dialog(message="是否使用系统测试值自动补偿" ("消息")) -> (T button?=w258:bool)  [unwired: 2 in]
                  }
                }
                n130 = global read "多参数全局变量.vi" "盐度显示"() -> (w253:cluster{"温度测量值":sgl, "测量值":sgl, "温度偏移修正值":sgl})
                n131 = Unbundle By Name(w253) -> ("测量值"=w252:sgl)
                n132 = property class="DigNum (严格)"(reference=w257) -> (reference out=w255:refnum<vi>, "Value"=w251:sgl)  [unwired: 1 in, 1 out]
                n133 = Select(t=w252, s=w254, f=w251) -> (s? t:f=w250:sgl)
                n134 = call "数字键盘.vi"("OldNumber"=w250) -> ("NewNumber"=w256:dbl)  [unwired: 1 in]
                n135 = property class="DigNum (严格)"(reference=w255, "Val(Sgnl)"=w256) -> ()  [unwired: 1 in, 2 out]
              }
              frame "Disabled", Default {
              }
            }
            n136 = call "Add State to Queue.vi"("State(s) In (\"\")"=w244) -> ("States Out"=w248:string)  [unwired: 14 in]
          }
          event "大气压力": Value Change {
            n137 = event-data() -> ("NewVal"=w261:sgl)  [unwired: 1 in, 3 out]
            n138 = global read "多参数全局变量.vi" "MB session in"() -> (w262:refnum<class "MB_Master.lvclass">)
            n139 = call "纳清DO_大气压力写入.vi"("数值"=w261, "MB session in"=w262) -> ()  [unwired: 8 in, 2 out]
            n140 = call "Add State to Queue.vi"("State(s) In (\"\")"=w260) -> ("States Out"=w264:string)  [unwired: 14 in]
          }
          event "盐度": Value Change {
            n141 = event-data() -> ("NewVal"=w266:sgl)  [unwired: 1 in, 5 out]
            n142 = global read "多参数全局变量.vi" "MB session in"() -> (w267:refnum<class "MB_Master.lvclass">)
            n143 = call "纳清DO_盐度写入.vi"("数值"=w266, "MB session in"=w267) -> ()  [unwired: 8 in, 2 out]
            n144 = call "Add State to Queue.vi"("State(s) In (\"\")"=w265) -> ("States Out"=w269:string)  [unwired: 14 in]
          }
          event "校准启动": Value Change {
            n145 = event-data() -> ()  [unwired: 1 in, 6 out]
            n146 = global read "多参数全局变量.vi" "校准运行状态"() -> (w271:T5)
            n147 = call "Add State to Queue.vi"("State(s) In (\"\")"=w276, "State(s) At Back (\"\")"="init: all\nCal: Place standard solution\n Cal: Calibration process\nidle" ("State(s) In (\"\")")) -> ("States Out"=w275:string)  [unwired: 13 in]
            n148 = Bundle By Name(cluster=w271, "DO"=TRUE) -> (w272:T5)
            n149 = global write "多参数全局变量.vi" "校准运行状态"(w272) -> ()
          }
          event "校准停止": Value Change {
            n150 = event-data() -> ()  [unwired: 1 in, 6 out]
            n151 = call "Add State to Queue.vi"("State(s) In (\"\")"="init: all\nCal: Over\nidle" ("State(s) In (\"\")")) -> ("States Out"=w278:string)  [unwired: 14 in]
          }
        }
      }
    }
  }
